vi "AD-DA .vi"() -> ()   [LabVIEW 2012]
panel:
  in  "设置CAN  DA输出":bool
  in  "CAN  AD-DA":T1={"AD0:"=0.0, "AD1:"=0.0, "AD2:"=0.0, "AD3:"=0.0, "DA0: "=5.0, "DA1: "=5.0}
  in  "电压/电流模式设置":enum16{"电压模式", "电流模式"}(ring)
  in  "保存":bool
  in  "设置DA输出模式":bool
  in  "CAN节点设置":u16=1
  in  "CAN断开":bool
  in  "CAN连接":bool
  out "CAN节点数":dbl
  in  "设置DA输出":bool
  in  "AD-DA":T2={"AD0:"=0.0, "AD1:"=0.0, "AD2:"=0.0, "AD3:"=0.0, "AD4:"=0.0, "AD5:"=0.0, "AD6:"=0.0, "AD7:"=0.0, "DA0: "=5.0, "DA1: "=5.0}
  out "CAN通讯状态":string
  out "当前速度":dbl
  in  "退出":bool
  in  "卡号选择":u16(ring) items=["0"]
  out "init":bool
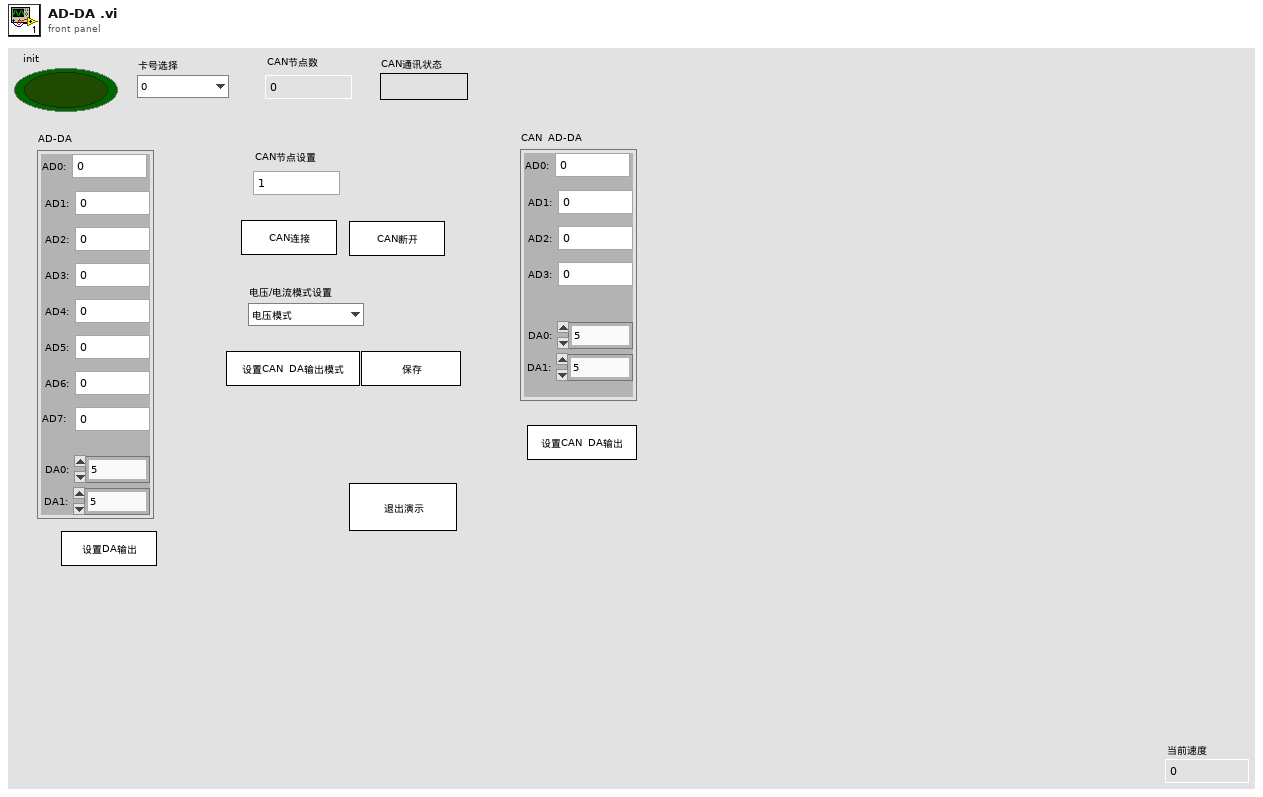
[diagram p1: front panel]
types:
  T1 = cluster{"AD0:":dbl, "AD1:":dbl, "AD2:":dbl, "AD3:":dbl, "DA0: ":dbl, "DA1: ":dbl}
  T2 = cluster{"AD0:":dbl, "AD1:":dbl, "AD2:":dbl, "AD3:":dbl, "AD4:":dbl, "AD5:":dbl, "AD6:":dbl, "AD7:":dbl, "DA0: ":dbl, "DA1: ":dbl}
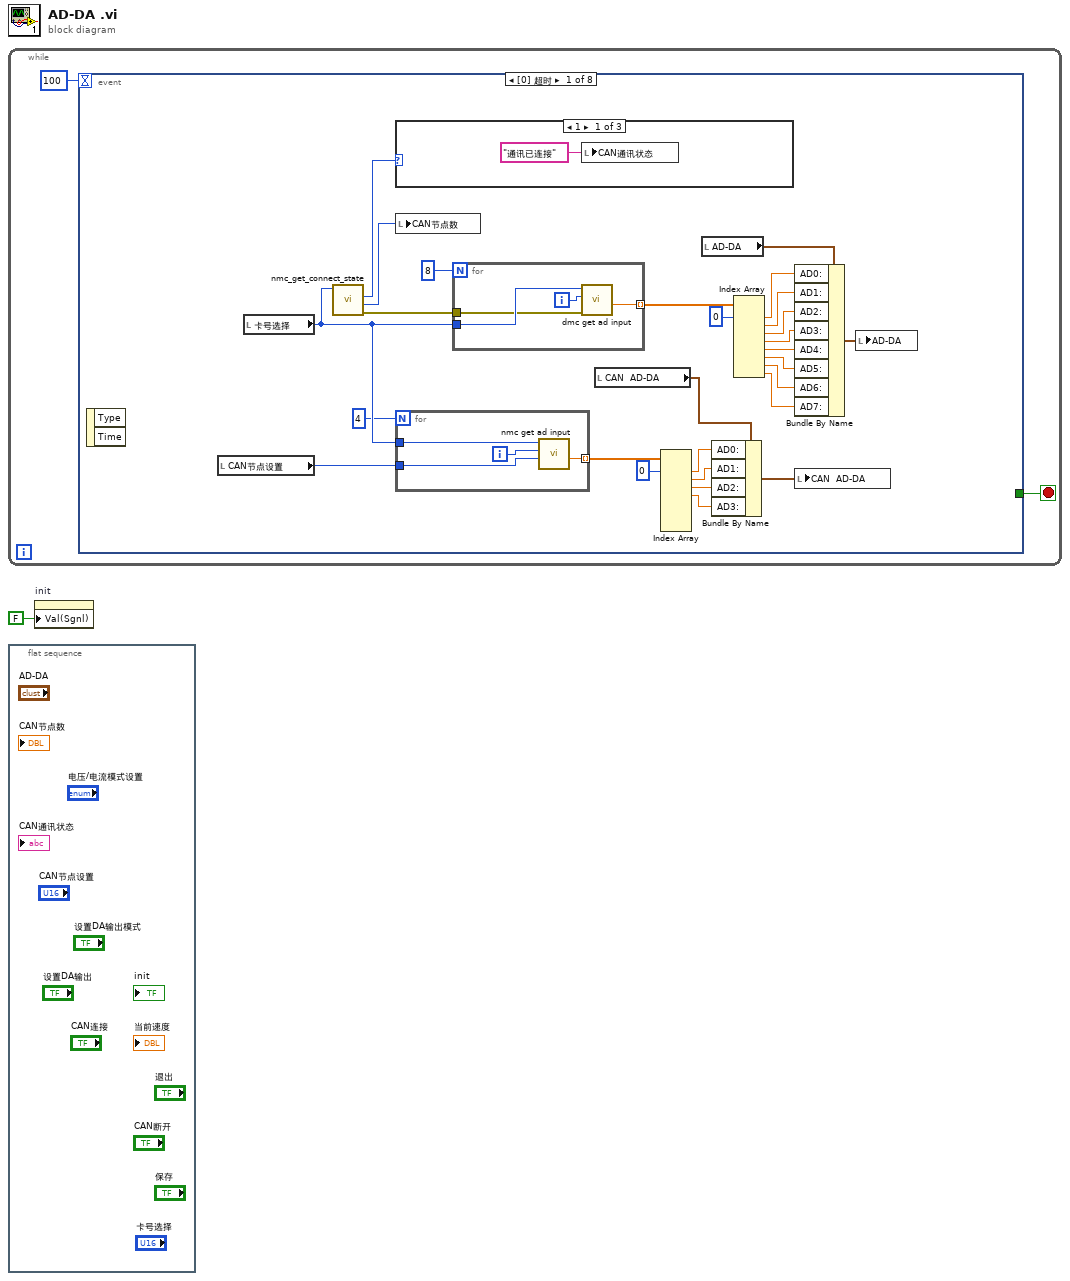
[diagram p0: block diagram]
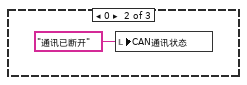
[diagram p2: hidden frame]
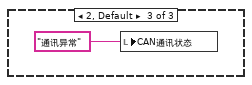
[diagram p3: hidden frame]
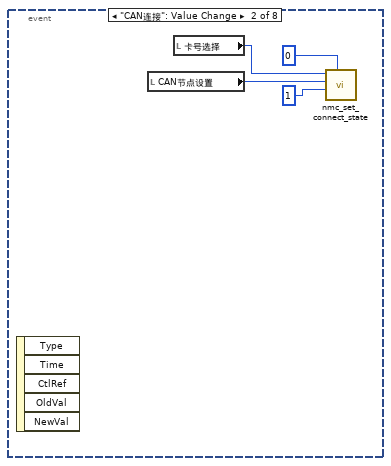
[diagram p4: hidden frame]
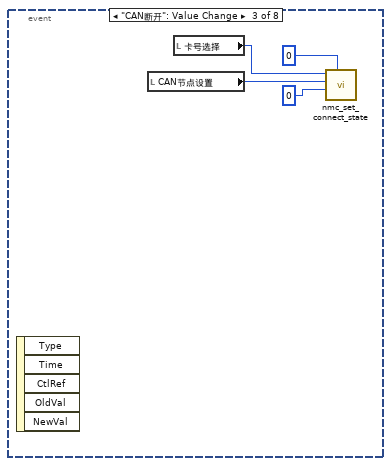
[diagram p5: hidden frame]
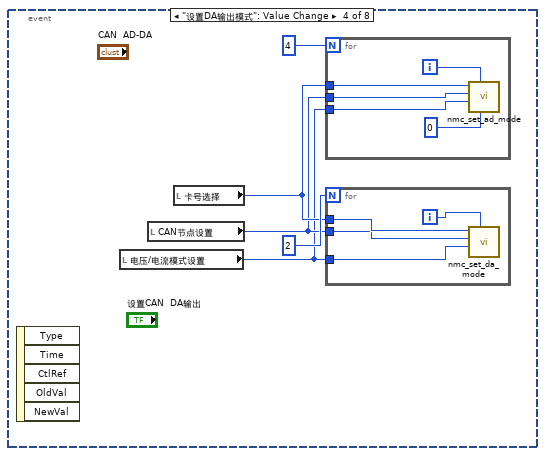
[diagram p6: hidden frame]
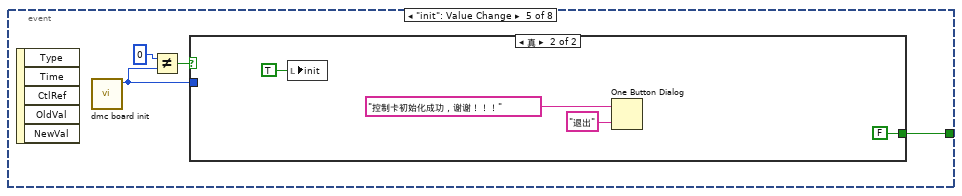
[diagram p7: hidden frame]
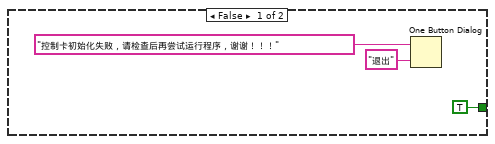
[diagram p8: hidden frame]
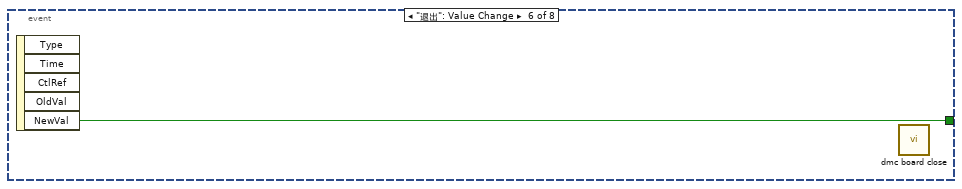
[diagram p9: hidden frame]
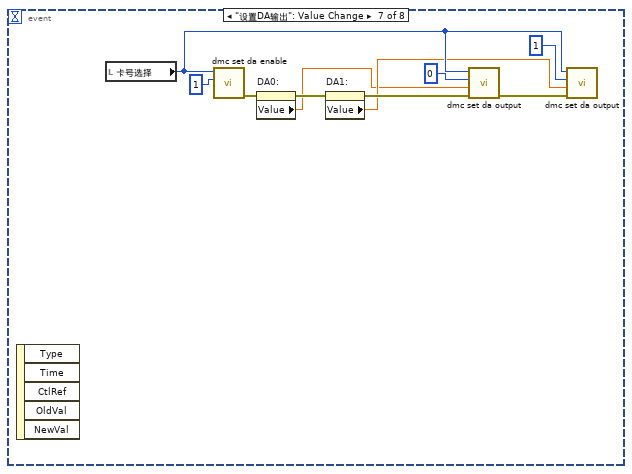
[diagram p10: hidden frame]
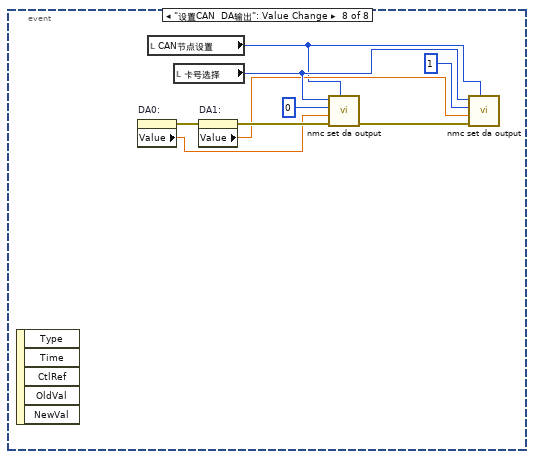
[diagram p11: hidden frame]
diagram:
  n1 = while {
    stop <- w3 stop-if-true
    n2 = event shown="[0] 超时" {
      selector: _ -> [_ _ _ _ _ _ _ _]
      dyn-events: _ -> [_ _ _ _ _ _ _ _]
      timeout: 100 -> [_ _ _ _ _ _ _ _]
      tunnel: [_ _ _ _ w66 w75 _ _] -> w3
      event Timeout {
        n3 = event-data() -> ()  [unwired: 1 in, 2 out]
        n4 = local read "CAN节点设置"() -> (w12:u16)
        n5 = local read "卡号选择"() -> (w14:u16)
        n6 = call "nmc_get_connect_state.vi"("CardNo"=w14) -> ("error out"=w17:errorcluster, "node 2"=w16:u16, "CAN states 2"=w15:u16)  [unwired: 7 in, 1 out]
        n7 = case shown="1" w15 {
          frame 1 {
            n8 = local write "CAN通讯状态"("通讯已连接" ("CAN通讯状态")) -> ()
          }
          frame 0 {
            n9 = local write "CAN通讯状态"("通讯已断开" ("CAN通讯状态")) -> ()
          }
          frame 2, Default {
            n10 = local write "CAN通讯状态"("通讯异常" ("CAN通讯状态")) -> ()
          }
        }
        n11 = local write "CAN节点数"(w16) -> ()
        n12 = for {
          N: 4 -> [_]
          tunnel: w14 -> [w34]
          tunnel: w12 -> [w32]
          tunnel: [w31] -> w10 mode=indexing
          i -> [w33]
          n13 = call "nmc get ad input.vi"("node"=w32, "channel"=w33, "CardNo"=w34) -> ("Vout out"=w31:dbl)  [unwired: 6 in, 2 out]
        }
        n14 = for {
          N: 8 -> [_]
          tunnel: w14 -> [w41]
          tunnel: [w39] -> w27 mode=indexing
          tunnel: w17 -> [w38]
          i -> [w40]
          n15 = call "dmc get ad input.vi"("error in (no error)"=w38, "channel"=w40, "CardNo"=w41) -> ("Vout out"=w39:dbl)  [unwired: 6 in, 2 out]
        }
        n16 = local read "CAN  AD-DA"() -> (w11:T1)
        n17 = Index Array(array=w10, index #1=0 ("索引")) -> (element #1=w8:dbl, element #2=w7:dbl, element #3=w6:dbl, element #4=w5:dbl)  [unwired: 7 in, 4 out]
        n18 = local read "AD-DA"() -> (w30:T2)
        n19 = Bundle By Name(cluster=w11, "AD0:"=w8, "AD1:"=w7, "AD2:"=w6, "AD3:"=w5) -> (w4:T1)
        n20 = Index Array(array=w27, index #1=0 ("索引")) -> (element #1=w25:dbl, element #2=w24:dbl, element #3=w23:dbl, element #4=w22:dbl, element #5=w21:dbl, element #6=w20:dbl, element #7=w19:dbl, element #8=w18:dbl)  [unwired: 7 in]
        n21 = Bundle By Name(cluster=w30, "AD0:"=w25, "AD1:"=w24, "AD2:"=w23, "AD3:"=w22, "AD4:"=w21, "AD5:"=w20, "AD6:"=w19, "AD7:"=w18) -> (w29:T2)
        n22 = local write "CAN  AD-DA"(w4) -> ()
        n23 = local write "AD-DA"(w29) -> ()
      }
      event "CAN连接": Value Change {
        n24 = event-data() -> ()  [unwired: 1 in, 5 out]
        n25 = local read "CAN节点设置"() -> (w42:u16)
        n26 = local read "卡号选择"() -> (w45:u16)
        n27 = call "nmc_set_connect_state.vi"("dd"=u16 0, "mode"=u16 1 ("node"), "node"=w42, "CardNo"=w45) -> ()  [unwired: 6 in, 2 out]
      }
      event "CAN断开": Value Change {
        n28 = event-data() -> ()  [unwired: 1 in, 5 out]
        n29 = local read "CAN节点设置"() -> (w46:u16)
        n30 = local read "卡号选择"() -> (w49:u16)
        n31 = call "nmc_set_connect_state.vi"("dd"=u16 0, "mode"=u16 0 ("node"), "node"=w46, "CardNo"=w49) -> ()  [unwired: 6 in, 2 out]
      }
      event "设置DA输出模式": Value Change {
        n32 = event-data() -> ()  [unwired: 1 in, 5 out]
        n33 = local read "电压/电流模式设置"() -> (w50:enum16{"电压模式", "电流模式"})
        n34 = local read "CAN节点设置"() -> (w51:u16)
        n35 = local read "卡号选择"() -> (w52:u16)
        n36 = for {
          N: 4 -> [_]
          tunnel: w52 -> [w63]
          tunnel: w51 -> [w62]
          tunnel: w50 -> [w61]
          i -> [w59]
          n37 = call "nmc_set_ad_mode.vi"("buffer_nums"=u16 0, "channel"=w59, "mode"=w61, "node"=w62, "CardNo"=w63) -> ()  [unwired: 5 in, 2 out]
        }
        n38 = for {
          N: 2 -> [_]
          tunnel: w52 -> [w58]
          tunnel: w51 -> [w57]
          tunnel: w50 -> [w56]
          i -> [w55]
          n39 = call "nmc_set_da_mode.vi"("channel"=w55, "mode"=w56, "node"=w57, "CardNo"=w58) -> ()  [unwired: 6 in, 2 out]
        }
      }
      event "init": Value Change {
        n40 = event-data() -> ()  [unwired: 1 in, 5 out]
        n41 = call "dmc board init.vi"() -> ("function return"=w65:i16)  [unwired: 10 in, 1 out]
        n42 = Not Equal?(x=0, y=w65) -> (x != y?=w67:bool)
        n43 = case shown="真" w67 {
          tunnel: [TRUE ("true") FALSE ("true")] -> w66
          tunnel: w65 -> [_ _]
          frame False {
            n44 = One Button Dialog(message="控制卡初始化失败，请检查后再尝试运行程序，谢谢！！！" ("消息"), button name ("OK")="退出" ("按钮名称（“确定”）")) -> ()  [unwired: 1 out]
          }
          frame True {
            n45 = local write "init"(TRUE ("init")) -> ()
            n46 = One Button Dialog(message="控制卡初始化成功，谢谢！！！" ("消息"), button name ("OK")="退出" ("按钮名称（“确定”）")) -> ()  [unwired: 1 out]
          }
        }
      }
      event "退出": Value Change {
        n47 = event-data() -> ("NewVal"=w75:bool)  [unwired: 1 in, 4 out]
        n48 = call "dmc board close.vi"() -> ()  [unwired: 10 in, 2 out]
      }
      event "设置DA输出": Value Change {
        n49 = event-data() -> ()  [unwired: 1 in, 5 out]
        n50 = local read "卡号选择"() -> (w79:u16)
        n51 = call "dmc set da enable.vi"("enable"=u16 1, "CardNo"=w79) -> ("error out"=w84:errorcluster)  [unwired: 8 in, 1 out]
        n52 = property on="DA0:" class="DigNum (严格)"(error in=w84) -> (error out=w83:errorcluster, "Value"=w77:dbl)  [unwired: 1 in, 1 out]
        n53 = property on="DA1:" class="DigNum (严格)"(error in=w83) -> (error out=w82:errorcluster, "Value"=w78:dbl)  [unwired: 1 in, 1 out]
        n54 = call "dmc set da output.vi"("error in (no error)"=w82, "Vout"=w77, "channel"=u16 0, "CardNo"=w79) -> ("error out"=w76:errorcluster)  [unwired: 6 in, 1 out]
        n55 = call "dmc set da output.vi"("error in (no error)"=w76, "Vout"=w78, "channel"=u16 1, "CardNo"=w79) -> ()  [unwired: 6 in, 2 out]
      }
      event "设置CAN  DA输出": Value Change {
        n56 = event-data() -> ()  [unwired: 1 in, 5 out]
        n57 = property on="DA0:" class="DigNum (严格)"() -> (error out=w94:errorcluster, "Value"=w88:dbl)  [unwired: 2 in, 1 out]
        n58 = local read "CAN节点设置"() -> (w86:u16)
        n59 = local read "卡号选择"() -> (w90:u16)
        n60 = property on="DA1:" class="DigNum (严格)"(error in=w94) -> (error out=w93:errorcluster, "Value"=w89:dbl)  [unwired: 1 in, 1 out]
        n61 = call "nmc set da output.vi"("node"=w86, "error in (no error)"=w93, "Vout"=w88, "channel"=u16 0, "CardNo"=w90) -> ("error out"=w87:errorcluster)  [unwired: 5 in, 1 out]
        n62 = call "nmc set da output.vi"("node"=w86, "error in (no error)"=w87, "Vout"=w89, "channel"=u16 1, "CardNo"=w90) -> ()  [unwired: 5 in, 2 out]
      }
    }
  }
  n63 = flat-sequence {
    frame #0 {
    }
  }
  n64 = property on="init" class="Bool (严格)"("Val(Sgnl)"=FALSE ("值(信号)")) -> ()  [unwired: 2 in, 2 out]
